vi "DELE.vi"(8 "error in (no error)":errorcluster, 10 "RemoteFileName":string, 11 "FTP in":refnum<class "FTP.lvclass">) -> (0 "error out":errorcluster, 3 "FTP out":refnum<class "FTP.lvclass">)   [LabVIEW 2020, in "FTP.lvlib" / "FTP.lvclass"]
uses:
  FTP.lvclass
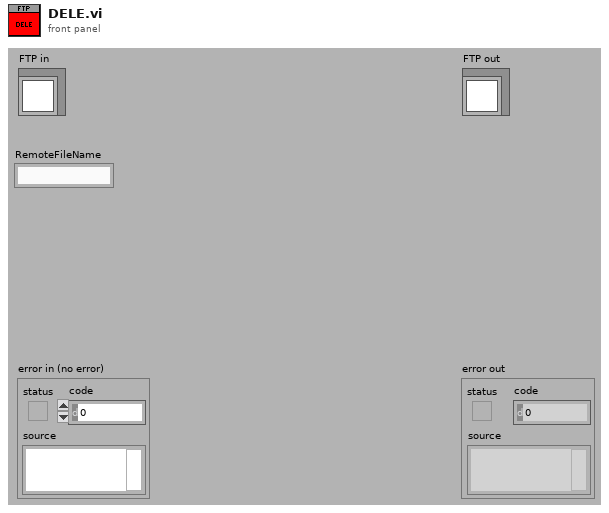
[diagram p1: front panel]
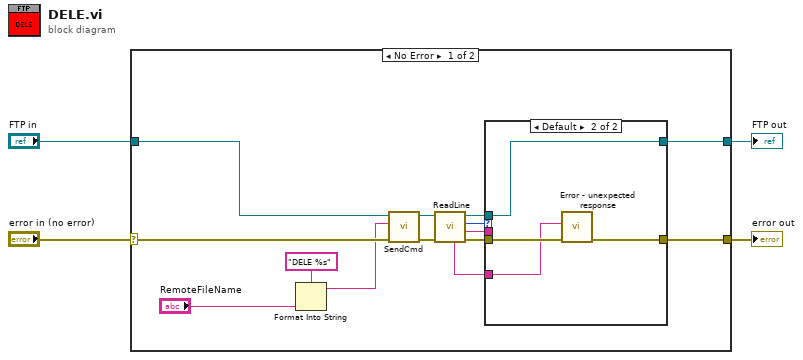
[diagram p0: block diagram]
diagram:
  n1 = case shown="No Error" "error in (no error)" {
    selector: "error in (no error)" -> [w12 w26]
    tunnel: [w11 w26] -> w3
    tunnel: [w10 w25] -> w1
    tunnel: "FTP in" -> [w9 w25]
    frame No Error {
      n2 = Format Into String(format string="DELE %s", "RemoteFileName") -> (resulting string=w7:string)  [unwired: 2 in, 1 out]
      n3 = call "SendCmd.vi"("error in (no error)"=w12, "cmd"=w7, "FTP in"=w9) -> ("error out"=w18:errorcluster, "FTP out"=w17:refnum<class "FTP.lvclass">)  [unwired: 7 in]
      n4 = call "ReadLine.vi"("error in (no error)"=w18, "FTP in"=w17) -> ("error out"=w14:errorcluster, "Line"=w13:string, "code"=w15:i32, "FTP out"=w16:refnum<class "FTP.lvclass">, "Full Line"=w5:string)  [unwired: 5 in]
      n5 = case shown="Default" w15 {
        tunnel: w16 -> [w20 w24]
        tunnel: w14 -> [w19 w23]
        tunnel: [w19 w22] -> w11
        tunnel: [w20 w24] -> w10
        tunnel: w13 -> [_ _]
        tunnel: w5 -> [_ w21]
        frame 200, 250 {
        }
        frame Default {
          n6 = call "Error - unexpected response.vi"("error in (no error)"=w23, "Full Response"=w21) -> ("error out"=w22:errorcluster)  [unwired: 9 in]
        }
      }
    }
    frame Error {
    }
  }
  "error out" <- w3
  "FTP out" <- w1
